vi "rollingArray.vi"   [LabVIEW 2014]
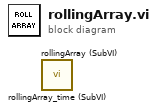
[diagram p0: block diagram]
diagram:
  n1 = call "rollingArray_time (SubVI).vi"() -> ()  [unwired: 11 in, 1 out]
  n2 = call "rollingArray (SubVI).vi"() -> ()  [unwired: 11 in, 1 out]
